vi "Implement When VIs.vi"(8 "error in (no error)":errorcluster, 10 "When VIs":path[](array[path]), 11 "Mock Class Generator In":refnum<class "Responsive Mock Class Generator.lvclass">) -> (0 "error out":errorcluster, 3 "Mock Class Generator Out":refnum<class "Responsive Mock Class Generator.lvclass">)   [LabVIEW 2020, in "Responsive Mock Class Generator.lvclass"]
uses:
  Responsive Mock Class Generator.lvclass
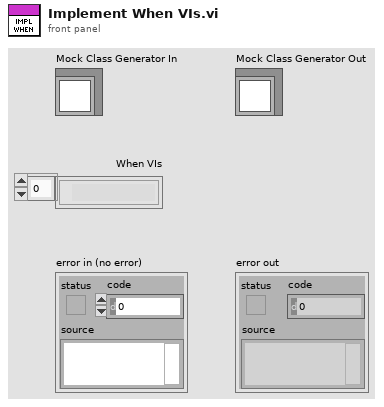
[diagram p1: front panel]
types:
  T1 = enum16{"Invalid Wire Rule", "Required", "Recommended", "Optional", "Dynamic Dispatch"}
  T2 = enum16{"Invalid Wire Rule", "Required", "Recommended", "Optional", "Dynamic Dispatch"}[]
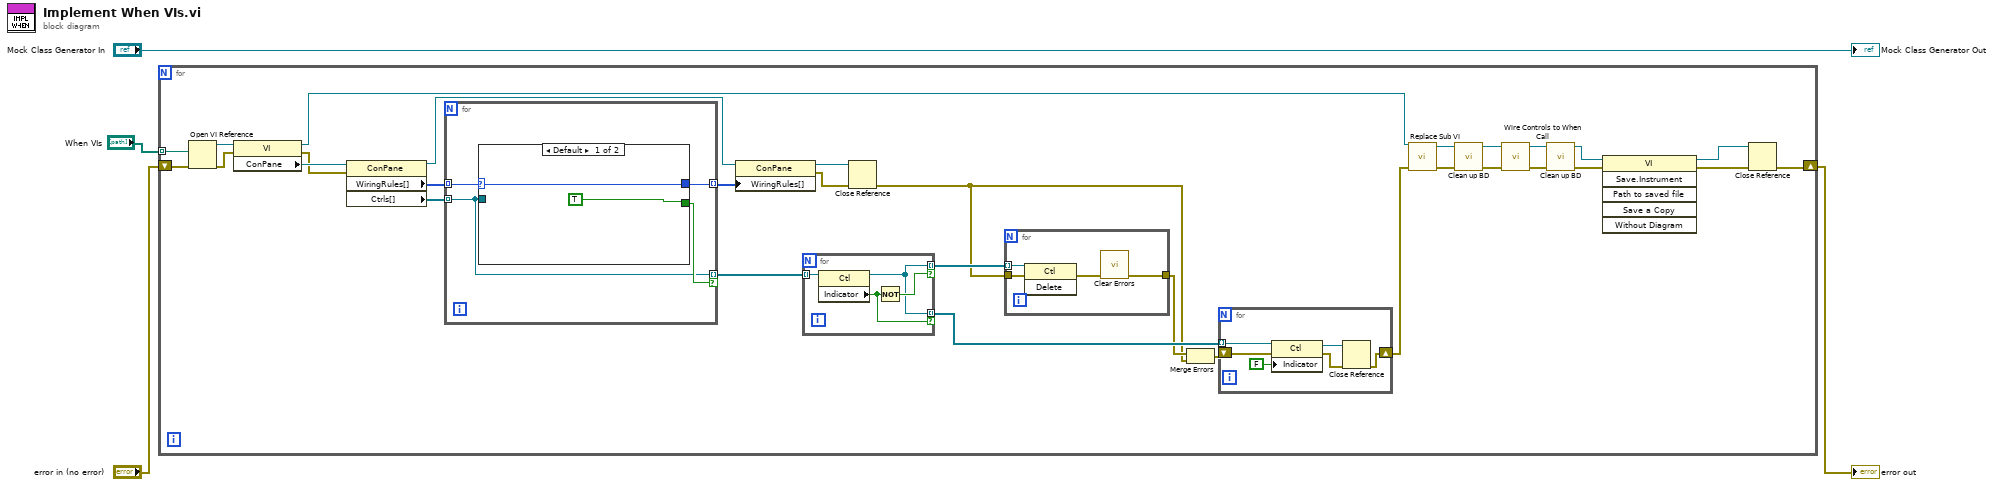
[diagram p0: block diagram]
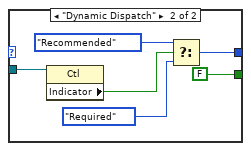
[diagram p2: hidden frame]
diagram:
  n1 = for {
    tunnel: "When VIs" -> [w35] mode=indexing
    shift-right: [w20] -> w1
    shift-left: "error in (no error)" -> [w34]
    n2 = Open VI Reference(vi path=w35, error in (no error)=w34) -> (vi reference=w33:refnum<vi>, error out=w25:errorcluster)  [unwired: 4 in]
    n3 = property class="VI"(reference=w33, error in=w25) -> (reference out=w21:refnum<vi>, error out=w22:errorcluster, "ConPane"=w32:refnum<vi>)
    n4 = property class="ConPane"(reference=w32, error in=w22) -> (reference out=w28:refnum<vi>, "WiringRules[]"=w31:T2, "Ctrls[]"=w29:refnum<vi>[])  [unwired: 1 out]
    n5 = for {
      tunnel: w31 -> [w39] mode=indexing
      tunnel: [w38] -> w30 mode=indexing
      tunnel: w29 -> [w36] mode=indexing
      tunnel: [w36] -> w27 mode=indexing if=w37
      n6 = case shown="Default" w39 {
        selector: w39 -> [w41 _]
        tunnel: [w41 w44] -> w38
        tunnel: [TRUE FALSE] -> w37
        tunnel: w36 -> [_ w45]
        frame Default {
        }
        frame "Dynamic Dispatch" {
          n7 = property class="Ctl"(reference=w45) -> ("Indicator"=w43:bool)  [unwired: 1 in, 2 out]
          n8 = Select(t=T1."Recommended" ("Wire Rule"), s=w43, f=T1."Required" ("Wire Rule")) -> (s? t:f=w44:T1)
        }
      }
    }
    n9 = property class="ConPane"(reference=w28, "WiringRules[]"=w30) -> (reference out=w12:refnum<vi>, error out=w24:errorcluster)  [unwired: 1 in]
    n10 = for {
      tunnel: [w59] -> w26 mode=indexing if=w60
      tunnel: w27 -> [w61] mode=indexing
      tunnel: [w59] -> w23 mode=indexing if=w58
      n11 = property class="Ctl"(reference=w61) -> (reference out=w59:refnum<vi>, "Indicator"=w58:bool)  [unwired: 1 in, 1 out]
      n12 = Not(x=w58) -> (.not. x?=w60:bool)
    }
    n13 = Close Reference(reference=w12, error in (no error)=w24) -> (error out=w13:errorcluster)
    n14 = for {
      tunnel: w26 -> [w57] mode=indexing
      tunnel: w13 -> [w55]
      tunnel: [w54] -> w15
      n15 = invoke class="Ctl" method="Delete"(reference=w57, error in=w55) -> (error out=w56:errorcluster)  [unwired: 1 in, 2 out]
      n16 = call <vilib>:"Clear Errors.vi"("error in (no error)"=w56) -> ("error out"=w54:errorcluster)  [unwired: 5 in, 1 out]
    }
    n17 = Merge Errors(w15, w13) -> (w14:errorcluster)
    n18 = for {
      tunnel: w23 -> [w53] mode=indexing
      shift-right: [w48] -> w19
      shift-left: w14 -> [w49]
      n19 = property class="Ctl"(reference=w53, error in=w49, "Indicator"=FALSE) -> (reference out=w50:refnum<vi>, error out=w51:errorcluster)
      n20 = Close Reference(reference=w50, error in (no error)=w51) -> (error out=w48:errorcluster)
    }
    n21 = call "Replace Sub VI.vi"("error in (no error)"=w19, "VI in"=w21) -> ("error out"=w18:errorcluster, "VI out"=w6:refnum<vi>)  [unwired: 8 in]
    n22 = call "Clean up BD.vi"("error in (no error)"=w18, "VI in"=w6) -> ("error out"=w7:errorcluster, "VI out"=w5:refnum<vi>)  [unwired: 8 in]
    n23 = call "Wire Controls to When Call.vi"("error in (no error)"=w7, "VI in"=w5) -> ("error out"=w9:errorcluster, "VI out"=w8:refnum<vi>)  [unwired: 8 in]
    n24 = call "Clean up BD.vi"("error in (no error)"=w9, "VI in"=w8) -> ("error out"=w11:errorcluster, "VI out"=w10:refnum<vi>)  [unwired: 8 in]
    n25 = invoke class="VI" method="Save.Instrument"(reference=w10, error in=w11) -> (reference out=w16:refnum<vi>, error out=w17:errorcluster)  [unwired: 4 in, 4 out]
    n26 = Close Reference(reference=w16, error in (no error)=w17) -> (error out=w20:errorcluster)
  }
  "error out" <- w1
  "Mock Class Generator Out" <- "Mock Class Generator In"
